vi "Get Module Info (FPGA Mode).vi"(8 "error in":errorcluster, 11 "Session in":refnum<k21>="localhost") -> (0 "error out":errorcluster, 2 "Module Information":T1[](array[typedef]) {"Module Code" format="%.0x"}, 3 "Session out":refnum<k21>="localhost")   [LabVIEW 2015]
uses:
  <vilib>/rvi/interface/nirviCloseFPGA/nirviCloseFPGA.xnode
  <vilib>/FPGAPlugInAG/Dynamic/niLvFpga_Close_Dynamic.vi
  <vilib>/rvi/interface/nirviMethod/nirviMethod.xnode
  <vilib>/FPGAPlugInAG/Dynamic/niLvFpga_Run_Dynamic.vi
  Controls/ModuleInformation.ctl
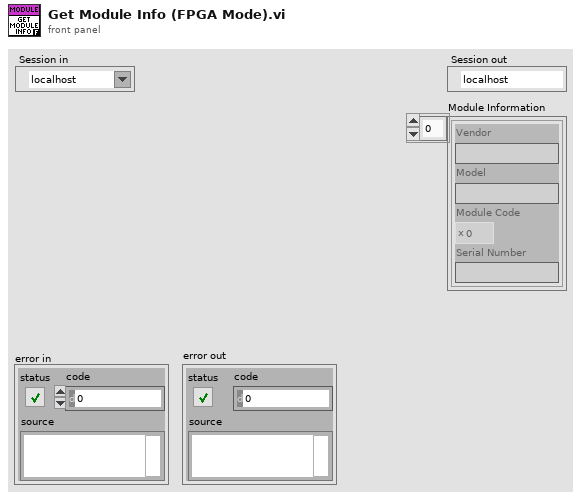
[diagram p1: front panel]
types:
  T1 = typedef "RT Management.lvlib/Module Detection.lvclass/ModuleInformation.ctl" = cluster{"Vendor":string, "Model":string, "Module Code":u32, "Serial Number":string}
  T2 = cluster{"Vendor and Module ID":u32, "Vendor Name":string, "Model Name":string, "Serial Number":u32}
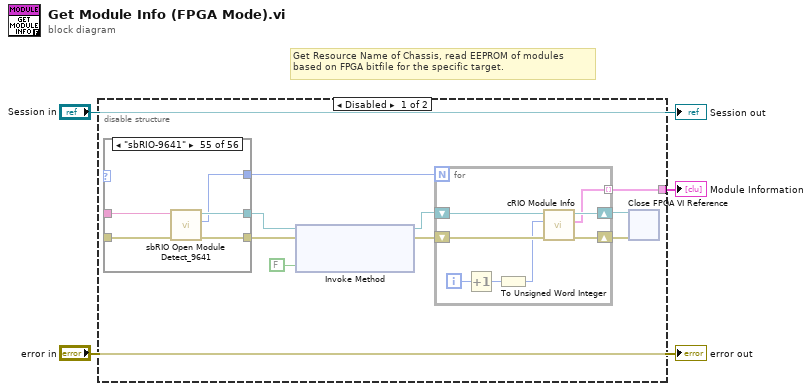
[diagram p0: block diagram]
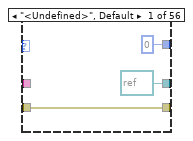
[diagram p2: hidden frame]
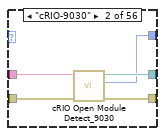
[diagram p3: hidden frame]
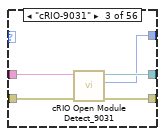
[diagram p4: hidden frame]
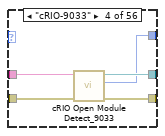
[diagram p5: hidden frame]
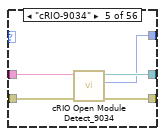
[diagram p6: hidden frame]
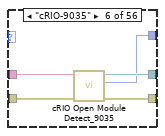
[diagram p7: hidden frame]
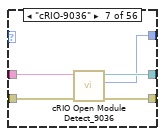
[diagram p8: hidden frame]
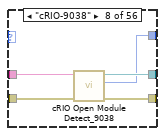
[diagram p9: hidden frame]
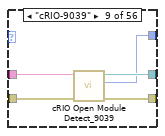
[diagram p10: hidden frame]
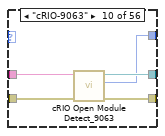
[diagram p11: hidden frame]
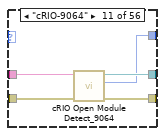
[diagram p12: hidden frame]
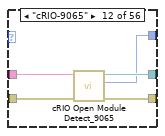
[diagram p13: hidden frame]
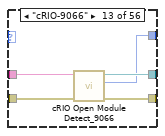
[diagram p14: hidden frame]
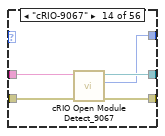
[diagram p15: hidden frame]
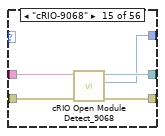
[diagram p16: hidden frame]
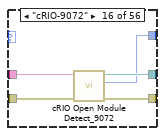
[diagram p17: hidden frame]
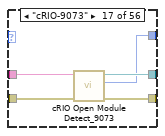
[diagram p18: hidden frame]
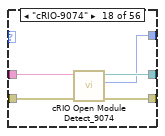
[diagram p19: hidden frame]
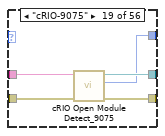
[diagram p20: hidden frame]
diagram:
  # "Get Resource Name of Chassis, read EEPROM of modules\nbased on FPGA bitfile for the specific target."
  n1 = disable-structure shown="Disabled" {
    disable-tunnel: [w4 _] -> w1
    frame Disabled {
      n2 = case shown="\"sbRIO-9641\"" {
        selector: _ -> [_ _ _ _ _ _ _ _ _ _ _ _ _ _ _ _ _ _ _ _ _ _ _ _ _ _ _ _ _ _ _ _ _ _ _ _ _ _ _ _ _ _ _ _ _ _ _ _ _ _ _ _ _ _ _ _]
        tunnel: _ -> [w15 w19 w24 w29 w34 w39 w44 w49 w54 w59 w64 w69 w74 w79 w84 w89 w94 w99 w104 w109 w114 w119 w124 w129 w134 w139 w144 w149 w154 w160 w165 w170 w175 w180 w185 w190 w195 w200 w205 w210 w213 w216 w221 w226 w229 w232 w237 w242 w245 w248 w253 w258 w261 w264 w269 w274]
        tunnel: [refnum<k20> refnum ("Refnum out") w18 w23 w28 w33 w38 w43 w48 w53 w58 w63 w68 w73 w78 w83 w88 w93 w98 w103 w108 w113 w118 w123 w128 w133 w138 w143 w148 w153 w159 w164 w169 w174 w179 w184 w189 w194 w199 w204 w209 refnum<k20> refnum ("Refnum out") refnum<k20> refnum ("Refnum out") w220 w225 refnum<k20> refnum ("Refnum out") refnum<k20> refnum ("Refnum out") w236 w241 refnum<k20> refnum ("Refnum out") refnum<k20> refnum ("Refnum out") w252 w257 refnum<k20> refnum ("Refnum out") refnum<k20> refnum ("Refnum out") w268 w273] -> w12
        tunnel: [w15 w20 w25 w30 w35 w40 w45 w50 w55 w60 w65 w70 w75 w80 w85 w90 w95 w100 w105 w110 w115 w120 w125 w130 w135 w140 w145 w150 w155 w158 w163 w168 w173 w178 w183 w188 w193 w198 w203 w208 w213 w216 w219 w224 w229 w232 w235 w240 w245 w248 w251 w256 w261 w264 w267 w272] -> w11
        tunnel: [0 ("slots") w17 w22 w27 w32 w37 w42 w47 w52 w57 w62 w67 w72 w77 w82 w87 w92 w97 w102 w107 w112 w117 w122 w127 w132 w137 w142 w147 w152 w157 w162 w167 w172 w177 w182 w187 w192 w197 w202 w207 0 ("slots") 0 ("slots") w218 w223 0 ("slots") 0 ("slots") w234 w239 0 ("slots") 0 ("slots") w250 w255 0 ("slots") 0 ("slots") w266 w271] -> w10
        tunnel: _ -> [_ w16 w21 w26 w31 w36 w41 w46 w51 w56 w61 w66 w71 w76 w81 w86 w91 w96 w101 w106 w111 w116 w121 w126 w131 w136 w141 w146 w151 w156 w161 w166 w171 w176 w181 w186 w191 w196 w201 w206 _ _ w217 w222 _ _ w233 w238 _ _ w249 w254 _ _ w265 w270]
        frame "<Undefined>", Default {
        }
        frame "cRIO-9030" {
          n3 = call "cRIO Open Module Detect_9030.vi"("error in (no error)"=w19, "RIO Device"=w16) -> ("error out"=w20:errorcluster, "slots"=w17:i32, "Refnum out"=w18:refnum<k20>)  [unwired: 7 in]
        }
        frame "cRIO-9031" {
          n4 = call "cRIO Open Module Detect_9031.vi"("error in (no error)"=w24, "RIO Device"=w21) -> ("error out"=w25:errorcluster, "slots"=w22:i32, "Refnum out"=w23:refnum<k20>)  [unwired: 7 in]
        }
        frame "cRIO-9033" {
          n5 = call "cRIO Open Module Detect_9033.vi"("error in (no error)"=w29, "RIO Device"=w26) -> ("error out"=w30:errorcluster, "slots"=w27:i32, "Refnum out"=w28:refnum<k20>)  [unwired: 7 in]
        }
        frame "cRIO-9034" {
          n6 = call "cRIO Open Module Detect_9034.vi"("error in (no error)"=w34, "RIO Device"=w31) -> ("error out"=w35:errorcluster, "slots"=w32:i32, "Refnum out"=w33:refnum<k20>)  [unwired: 7 in]
        }
        frame "cRIO-9035" {
          n7 = call "cRIO Open Module Detect_9035.vi"("error in"=w39, "RIO Device"=w36) -> ("error out"=w40:errorcluster, "slots"=w37:i32, "Refnum out"=w38:refnum<k20>)  [unwired: 7 in]
        }
        frame "cRIO-9036" {
          n8 = call "cRIO Open Module Detect_9036.vi"("error in"=w44, "RIO Device"=w41) -> ("error out"=w45:errorcluster, "slots"=w42:i32, "Refnum out"=w43:refnum<k20>)  [unwired: 7 in]
        }
        frame "cRIO-9038" {
          n9 = call "cRIO Open Module Detect_9038.vi"("error in (no error)"=w49, "RIO Device"=w46) -> ("error out"=w50:errorcluster, "slots"=w47:i32, "Refnum out"=w48:refnum<k20>)  [unwired: 7 in]
        }
        frame "cRIO-9039" {
          n10 = call "cRIO Open Module Detect_9039.vi"("error in"=w54, "RIO Device"=w51) -> ("error out"=w55:errorcluster, "slots"=w52:i32, "Refnum out"=w53:refnum<k20>)  [unwired: 7 in]
        }
        frame "cRIO-9063" {
          n11 = call "cRIO Open Module Detect_9063.vi"("error in"=w59, "RIO Device"=w56) -> ("error out"=w60:errorcluster, "slots"=w57:i32, "Refnum out"=w58:refnum<k20>)  [unwired: 7 in]
        }
        frame "cRIO-9064" {
          n12 = call "cRIO Open Module Detect_9064.vi"("error in"=w64, "RIO Device"=w61) -> ("error out"=w65:errorcluster, "slots"=w62:i32, "Refnum out"=w63:refnum<k20>)  [unwired: 7 in]
        }
        frame "cRIO-9065" {
          n13 = call "cRIO Open Module Detect_9065.vi"("error in"=w69, "RIO Device"=w66) -> ("error out"=w70:errorcluster, "slots"=w67:i32, "Refnum out"=w68:refnum<k20>)  [unwired: 7 in]
        }
        frame "cRIO-9066" {
          n14 = call "cRIO Open Module Detect_9066.vi"("error in (no error)"=w74, "RIO Device"=w71) -> ("error out"=w75:errorcluster, "slots"=w72:i32, "Refnum out"=w73:refnum<k20>)  [unwired: 7 in]
        }
        frame "cRIO-9067" {
          n15 = call "cRIO Open Module Detect_9067.vi"("error in (no error)"=w79, "RIO Device"=w76) -> ("error out"=w80:errorcluster, "slots"=w77:i32, "Refnum out"=w78:refnum<k20>)  [unwired: 7 in]
        }
        frame "cRIO-9068" {
          n16 = call "cRIO Open Module Detect_9068.vi"("error in"=w84, "RIO Device"=w81) -> ("error out"=w85:errorcluster, "slots"=w82:i32, "Refnum out"=w83:refnum<k20>)  [unwired: 7 in]
        }
        frame "cRIO-9072" {
          n17 = call "cRIO Open Module Detect_9072.vi"("error in (no error)"=w89, "RIO Device"=w86) -> ("error out"=w90:errorcluster, "slots"=w87:i32, "Refnum out"=w88:refnum<k20>)  [unwired: 7 in]
        }
        frame "cRIO-9073" {
          n18 = call "cRIO Open Module Detect_9073.vi"("error in (no error)"=w94, "RIO Device"=w91) -> ("error out"=w95:errorcluster, "slots"=w92:i32, "Refnum out"=w93:refnum<k20>)  [unwired: 7 in]
        }
        frame "cRIO-9074" {
          n19 = call "cRIO Open Module Detect_9074.vi"("error in (no error)"=w99, "RIO Device"=w96) -> ("error out"=w100:errorcluster, "slots"=w97:i32, "Refnum out"=w98:refnum<k20>)  [unwired: 7 in]
        }
        frame "cRIO-9075" {
          n20 = call "cRIO Open Module Detect_9075.vi"("error in (no error)"=w104, "RIO Device"=w101) -> ("error out"=w105:errorcluster, "slots"=w102:i32, "Refnum out"=w103:refnum<k20>)  [unwired: 7 in]
        }
        frame "cRIO-9076" {
          n21 = call "cRIO Open Module Detect_9076.vi"("error in (no error)"=w109, "RIO Device"=w106) -> ("error out"=w110:errorcluster, "slots"=w107:i32, "Refnum out"=w108:refnum<k20>)  [unwired: 7 in]
        }
        frame "cRIO-9081" {
          n22 = call "cRIO Open Module Detect_9081.vi"("error in (no error)"=w114, "RIO Device"=w111) -> ("error out"=w115:errorcluster, "slots"=w112:i32, "Refnum out"=w113:refnum<k20>)  [unwired: 7 in]
        }
        frame "cRIO-9082" {
          n23 = call "cRIO Open Module Detect_9082.vi"("error in (no error)"=w119, "RIO Device"=w116) -> ("error out"=w120:errorcluster, "slots"=w117:i32, "Refnum out"=w118:refnum<k20>)  [unwired: 7 in]
        }
        frame "cRIO-9101" {
          n24 = call "cRIO Open Module Detect_9101.vi"("error in (no error)"=w124, "RIO Device"=w121) -> ("error out"=w125:errorcluster, "slots"=w122:i32, "Refnum out"=w123:refnum<k20>)  [unwired: 7 in]
        }
        frame "cRIO-9102" {
          n25 = call "cRIO Open Module Detect_9102.vi"("error in (no error)"=w129, "RIO Device"=w126) -> ("error out"=w130:errorcluster, "slots"=w127:i32, "Refnum out"=w128:refnum<k20>)  [unwired: 7 in]
        }
        frame "cRIO-9103" {
          n26 = call "cRIO Open Module Detect_9103.vi"("error in (no error)"=w134, "RIO Device"=w131) -> ("error out"=w135:errorcluster, "slots"=w132:i32, "Refnum out"=w133:refnum<k20>)  [unwired: 7 in]
        }
        frame "cRIO-9104" {
          n27 = call "cRIO Open Module Detect_9104.vi"("error in (no error)"=w139, "RIO Device"=w136) -> ("error out"=w140:errorcluster, "slots"=w137:i32, "Refnum out"=w138:refnum<k20>)  [unwired: 7 in]
        }
        frame "cRIO-9111" {
          n28 = call "cRIO Open Module Detect_9111.vi"("error in (no error)"=w144, "RIO Device"=w141) -> ("error out"=w145:errorcluster, "slots"=w142:i32, "Refnum out"=w143:refnum<k20>)  [unwired: 7 in]
        }
        frame "cRIO-9112" {
          n29 = call "cRIO Open Module Detect_9112.vi"("error in (no error)"=w149, "RIO Device"=w146) -> ("error out"=w150:errorcluster, "slots"=w147:i32, "Refnum out"=w148:refnum<k20>)  [unwired: 7 in]
        }
        frame "cRIO-9113" {
          n30 = call "cRIO Open Module Detect_9113.vi"("error in (no error)"=w154, "RIO Device"=w151) -> ("error out"=w155:errorcluster, "slots"=w152:i32, "Refnum out"=w153:refnum<k20>)  [unwired: 7 in]
        }
        frame "cRIO-9114" {
          n31 = call "cRIO Open Module Detect_9114.vi"("error in (no error)"=w160, "RIO Device"=w156) -> ("error out"=w158:errorcluster, "slots"=w157:i32, "Refnum out"=w159:refnum<k20>)  [unwired: 7 in]
        }
        frame "cRIO-9116" {
          n32 = call "cRIO Open Module Detect_9116.vi"("error in (no error)"=w165, "RIO Device"=w161) -> ("error out"=w163:errorcluster, "slots"=w162:i32, "Refnum out"=w164:refnum<k20>)  [unwired: 7 in]
        }
        frame "cRIO-9118" {
          n33 = call "cRIO Open Module Detect_9118.vi"("error in (no error)"=w170, "RIO Device"=w166) -> ("error out"=w168:errorcluster, "slots"=w167:i32, "Refnum out"=w169:refnum<k20>)  [unwired: 7 in]
        }
        frame "NI 9146" {
          n34 = call "Ethernet RIO Open Module Detect_9146.vi"("error in"=w175, "RIO Device"=w171) -> ("error out"=w173:errorcluster, "slots"=w172:i32, "Refnum out"=w174:refnum<k20>)  [unwired: 7 in]
        }
        frame "NI 9147" {
          n35 = call "Ethernet RIO Open Module Detect_9147.vi"("error in (no error)"=w180, "RIO Device"=w176) -> ("error out"=w178:errorcluster, "slots"=w177:i32, "Refnum out"=w179:refnum<k20>)  [unwired: 7 in]
        }
        frame "NI 9148" {
          n36 = call "Ethernet RIO Open Module Detect_9148.vi"("error in (no error)"=w185, "RIO Device"=w181) -> ("error out"=w183:errorcluster, "slots"=w182:i32, "Refnum out"=w184:refnum<k20>)  [unwired: 7 in]
        }
        frame "NI 9149" {
          n37 = call "Ethernet RIO Open Module Detect_9149.vi"("error in (no error)"=w190, "RIO Device"=w186) -> ("error out"=w188:errorcluster, "slots"=w187:i32, "Refnum out"=w189:refnum<k20>)  [unwired: 7 in]
        }
        frame "NI 9154" {
          n38 = call "MXI-Express RIO Open Module Detect_9154.vi"("error in"=w195, "RIO Device"=w191) -> ("error out"=w193:errorcluster, "slots"=w192:i32, "Refnum out"=w194:refnum<k20>)  [unwired: 7 in]
        }
        frame "NI 9155" {
          n39 = call "MXI-Express RIO Open Module Detect_9155.vi"("error in"=w200, "RIO Device"=w196) -> ("error out"=w198:errorcluster, "slots"=w197:i32, "Refnum out"=w199:refnum<k20>)  [unwired: 7 in]
        }
        frame "NI 9157" {
          n40 = call "MXI-Express RIO Open Module Detect_9157.vi"("error in (no error)"=w205, "RIO Device"=w201) -> ("error out"=w203:errorcluster, "slots"=w202:i32, "Refnum out"=w204:refnum<k20>)  [unwired: 7 in]
        }
        frame "NI 9159" {
          n41 = call "MXI-Express RIO Open Module Detect_9159.vi"("error in (no error)"=w210, "RIO Device"=w206) -> ("error out"=w208:errorcluster, "slots"=w207:i32, "Refnum out"=w209:refnum<k20>)  [unwired: 7 in]
        }
        frame "myRIO-1900" {
        }
        frame "myRIO-1950" {
        }
        frame "sbRIO-9601" {
          n42 = call "sbRIO Open Module Detect_9601.vi"("error in (no error)"=w221, "RIO Device"=w217) -> ("error out"=w219:errorcluster, "slots"=w218:i32, "Refnum out"=w220:refnum<k20>)  [unwired: 7 in]
        }
        frame "sbRIO-9602" {
          n43 = call "sbRIO Open Module Detect_9602.vi"("error in (no error)"=w226, "RIO Device"=w222) -> ("error out"=w224:errorcluster, "slots"=w223:i32, "Refnum out"=w225:refnum<k20>)  [unwired: 7 in]
        }
        frame "sbRIO-9605" {
        }
        frame "sbRIO-9606" {
        }
        frame "sbRIO-9611" {
          n44 = call "sbRIO Open Module Detect_9611.vi"("error in"=w237, "RIO Device"=w233) -> ("error out"=w235:errorcluster, "slots"=w234:i32, "Refnum out"=w236:refnum<k20>)  [unwired: 7 in]
        }
        frame "sbRIO-9612" {
          n45 = call "sbRIO Open Module Detect_9612.vi"("error in"=w242, "RIO Device"=w238) -> ("error out"=w240:errorcluster, "slots"=w239:i32, "Refnum out"=w241:refnum<k20>)  [unwired: 7 in]
        }
        frame "sbRIO-9623" {
        }
        frame "sbRIO-9626" {
        }
        frame "sbRIO-9631" {
          n46 = call "sbRIO Open Module Detect_9631.vi"("error in"=w253, "RIO Device"=w249) -> ("error out"=w251:errorcluster, "slots"=w250:i32, "Refnum out"=w252:refnum<k20>)  [unwired: 7 in]
        }
        frame "sbRIO-9632" {
          n47 = call "sbRIO Open Module Detect_9632.vi"("error in"=w258, "RIO Device"=w254) -> ("error out"=w256:errorcluster, "slots"=w255:i32, "Refnum out"=w257:refnum<k20>)  [unwired: 7 in]
        }
        frame "sbRIO-9633" {
        }
        frame "sbRIO-9636" {
        }
        frame "sbRIO-9641" {
          n48 = call "sbRIO Open Module Detect_9641.vi"("error in"=w269, "RIO Device"=w265) -> ("error out"=w267:errorcluster, "slots"=w266:i32, "Refnum out"=w268:refnum<k20>)  [unwired: 7 in]
        }
        frame "sbRIO-9642" {
          n49 = call "sbRIO Open Module Detect_9642.vi"("error in"=w274, "RIO Device"=w270) -> ("error out"=w272:errorcluster, "slots"=w271:i32, "Refnum out"=w273:refnum<k20>)  [unwired: 7 in]
        }
      }
      n50 = xnode "Invoke Method"("FPGA VI Reference In"=w12, "error in"=w11, "Wait Until Done (F)"=FALSE) -> ("FPGA VI Reference Out"=w6:refnum<k20>, "error out"=w7:errorcluster)
      n51 = for {
        N: w10 -> [_]
        shift-right: [w279] -> w9
        shift-left: w6 -> [w282]
        shift-right: [w280] -> w8
        shift-left: w7 -> [w281]
        tunnel: [w275] -> w4 mode=indexing
        i -> [w278]
        n52 = Increment(x=w278) -> (x+1=w277:i32)
        n53 = To Unsigned Word Integer(number=w277) -> (unsigned 16bit integer=w276:u16)
        n54 = call "cRIO Module Info.vi"("error in"=w281, "Module"=w276, "Refnum in"=w282) -> ("error out"=w280:errorcluster, "cRIO Module Info"=w275:T2, "Refnum out"=w279:refnum<k20>)  [unwired: 6 in]
      }
      n55 = xnode "Close FPGA VI Reference"("FPGA VI Reference In"=w9, "error in"=w8) -> ()  [unwired: 1 out]
    }
    frame Enabled {
    }
  }
  "Module Information" <- w1
  "Session out" <- "Session in"
  "error out" <- "error in"
